vi "Acquisition State Machine.vi"(0 "Acquire":bool, 5 "Frames to Acquire":u32, 7 "Line Scan":bool, 9 "Line Scan Height":u32, 11 "Cancel Acq":bool, 12 "Enables":T1={"Enables Valid"=FALSE, "Frame Valid"=FALSE, "Line Valid"=FALSE, "Data Valid"=TRUE}) -> (4 "Acq In Progress":bool, 6 "Num Clocks Per Line":u32, 8 "Num Lines Per Frame":u32, 10 "Num Frames Acq'd":u32, 14 "Acquiring":bool, 15 "Capture Cycle":bool)   [LabVIEW 2014]
doc: "The Acquisition State Machine VI monitors its acquisition control inputs and tracks the state of the Camera Link enable signals to determine when pixel data should be captured and when it should be ignored, as indicated by the <B>Capture Cycle</B> output. The VI supports finite and continuous acquisitions for both area and line scan cameras. This VI is intended to run within a single-cycle timed loop.\n\nNote that the <B>Capture Cycle</B> output is delayed by two clock cycles relative to the <B>Enables</B> input. Also, this VI does not support cameras that change FVAL while LVAL is asserted. However, FVAL and LVAL are allowed to change at the same time. Open the VI for more documentation."
panel:
  # "Refer to the Context Help for a\ndescription of the controls and\nindicators of this VI."
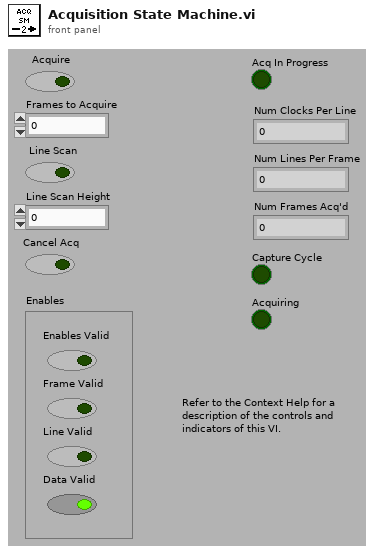
[diagram p1: front panel]
types:
  T1 = cluster{"Enables Valid":bool, "Frame Valid":bool, "Line Valid":bool, "Data Valid":bool}
  T2 = enum16{"Idle", "WaitForBlanking", "WaitForStartOfFrame", "WaitForEndOfFrame"}
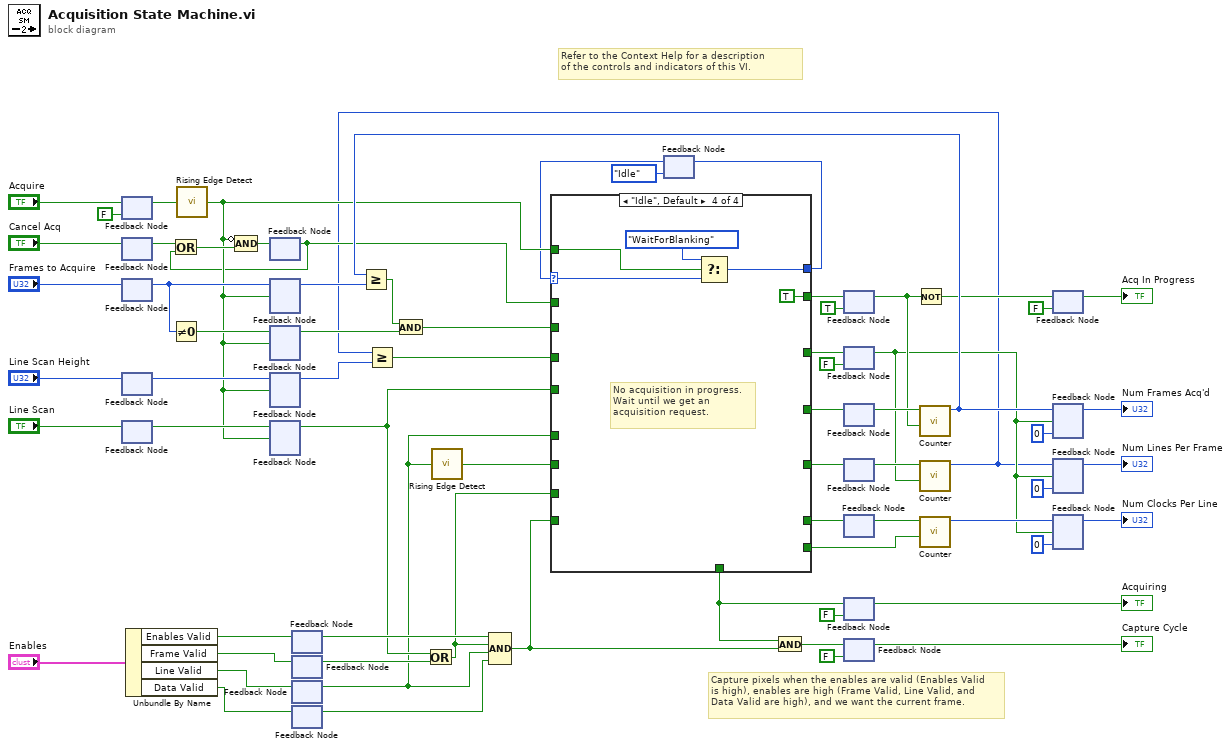
[diagram p0: block diagram]
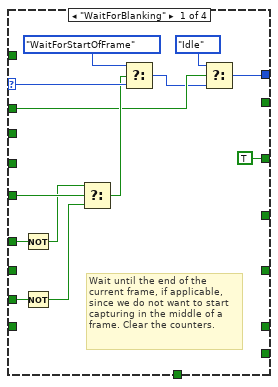
[diagram p2: hidden frame]
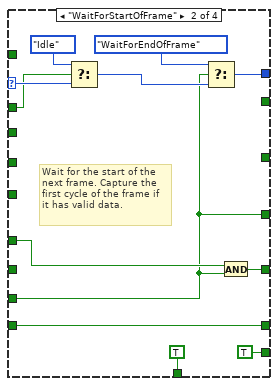
[diagram p3: hidden frame]
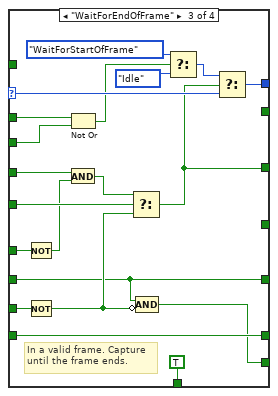
[diagram p4: hidden frame]
diagram:
  # "Refer to the Context Help for a description\nof the controls and indicators of this VI."
  # "Capture pixels when the enables are valid (Enables Valid\nis high), enables are high (Frame Valid, Line Valid, and\nData Valid are high), and we want the current frame."
  n1 = feedback #1(FALSE ("Acquire")) -> (w39:bool)
  n2 = feedback-in #1("Acquire") -> ()
  n3 = feedback #2() -> (w41:bool)  [unwired: 1 in]
  n4 = feedback-in #2("Cancel Acq") -> ()
  n5 = feedback #3() -> (w51:u32)  [unwired: 1 in]
  n6 = feedback-in #3("Frames to Acquire") -> ()
  n7 = feedback #4() -> (w36:u32)  [unwired: 1 in]
  n8 = feedback-in #4("Line Scan Height") -> ()
  n9 = feedback #5() -> (w34:bool)  [unwired: 1 in]
  n10 = feedback-in #5("Line Scan") -> ()
  n11 = Unbundle By Name("Enables") -> ("Enables Valid"=w29:bool, "Frame Valid"=w28:bool, "Line Valid"=w27:bool, "Data Valid"=w26:bool)
  n12 = Not Equal To 0?(x=w51) -> (x != 0?=w63:bool)
  n13 = call "Rising Edge Detect.vi"("Input"=w39) -> ("Pulse"=w33:bool)  [unwired: 4 in]
  n14 = feedback #6() -> (w25:bool)  [unwired: 1 in]
  n15 = Or(x=w41, y=w25) -> (x .or. y?=w43:bool)
  n16 = Compound Arithmetic op=AND(invert w33, w43) -> (w42:bool)
  n17 = feedback-in #6(w42) -> ()
  n18 = feedback #7() -> (w59:u32)  [unwired: 1 in]
  n19 = feedback-in #7(w51, w33) -> ()
  n20 = feedback #8() -> (w60:bool)  [unwired: 1 in]
  n21 = feedback-in #8(w63, w33) -> ()
  n22 = feedback #9() -> (w17:u32)  [unwired: 1 in]
  n23 = feedback-in #9(w36, w33) -> ()
  n24 = feedback #10() -> (w19:bool)  [unwired: 1 in]
  n25 = feedback-in #10(w34, w33) -> ()
  n26 = feedback #11() -> (w48:bool)  [unwired: 1 in]
  n27 = feedback-in #11(w29) -> ()
  n28 = feedback #12() -> (w32:bool)  [unwired: 1 in]
  n29 = feedback-in #12(w28) -> ()
  n30 = feedback #13() -> (w16:bool)  [unwired: 1 in]
  n31 = feedback-in #13(w27) -> ()
  n32 = feedback #14() -> (w46:bool)  [unwired: 1 in]
  n33 = feedback-in #14(w26) -> ()
  n34 = Or(x=w19, y=w32) -> (x .or. y?=w31:bool)
  n35 = call "Rising Edge Detect.vi"("Input"=w16) -> ("Pulse"=w40:bool)  [unwired: 4 in]
  n36 = Compound Arithmetic op=AND(w48, w31, w16, w46) -> (w47:bool)
  n37 = feedback #15(T2."Idle") -> (w23:T2)
  n38 = feedback #16(TRUE) -> (w20:bool)
  n39 = feedback #17(FALSE) -> (w6:bool)
  n40 = feedback #18() -> (w67:bool)  [unwired: 1 in]
  n41 = feedback #19() -> (w68:bool)  [unwired: 1 in]
  n42 = feedback #20() -> (w55:bool)  [unwired: 1 in]
  n43 = feedback #21(FALSE) -> (→"Acquiring":bool)
  n44 = feedback #22(FALSE) -> (→"Capture Cycle":bool)
  n45 = Not(x=w20) -> (.not. x?=w21:bool)
  n46 = call "Counter.vi"("Restart?"=w20, "Increment?"=w67) -> ("Count"=w62:u32)  [unwired: 9 in]
  n47 = Greater Or Equal?(x=w62, y=w59) -> (x >= y?=w61:bool)
  n48 = And(x=w61, y=w60) -> (x .and. y?=w18:bool)
  n49 = call "Counter.vi"("Restart?"=w6, "Increment?"=w68) -> ("Count"=w1:u32)  [unwired: 9 in]
  n50 = Greater Or Equal?(x=w1, y=w17) -> (x >= y?=w5:bool)
  n51 = case shown="\"Idle\", Default" w23 {
    selector: w23 -> [w82 w94 w113 w118]
    tunnel: [w75 w90 w114 w119] -> w22
    tunnel: [_ TRUE TRUE _] -> w3
    tunnel: w33 -> [_ _ _ w117]
    tunnel: w31 -> [w80 w83 w98 _]
    tunnel: [_ w85 w95 _] -> w69
    tunnel: [_ w83 _ _] -> w66
    tunnel: [TRUE _ w109 _] -> w8
    tunnel: w18 -> [_ _ w100 _]
    tunnel: [_ _ _ TRUE] -> w58
    tunnel: [_ w86 w111 _] -> w54
    tunnel: w47 -> [_ w86 w111 _]
    tunnel: [_ TRUE w97 _] -> w53
    tunnel: w40 -> [_ _ w95 _]
    tunnel: w5 -> [_ _ w102 _]
    tunnel: w19 -> [w81 _ w106 _]
    tunnel: w25 -> [w77 w89 w101 _]
    tunnel: w16 -> [w72 w84 w105 _]
    frame "WaitForBlanking" {
      # "Wait until the end of the\ncurrent frame, if applicable,\nsince we do not want to start\ncapturing in the middle of a\nframe. Clear the counters."
      n52 = Not(x=w72) -> (.not. x?=w71:bool)
      n53 = Not(x=w80) -> (.not. x?=w78:bool)
      n54 = Select(t=w71, s=w81, f=w78) -> (s? t:f=w79:bool)
      n55 = Select(t=T2."WaitForStartOfFrame", s=w79, f=w82) -> (s? t:f=w76:T2)
      n56 = Select(t=T2."Idle", s=w77, f=w76) -> (s? t:f=w75:T2)
    }
    frame "WaitForStartOfFrame" {
      # "Wait for the start of the\nnext frame. Capture the\nfirst cycle of the frame if\nit has valid data."
      n57 = Select(t=T2."Idle", s=w89, f=w94) -> (s? t:f=w91:T2)
      n58 = Select(t=T2."WaitForEndOfFrame", s=w83, f=w91) -> (s? t:f=w90:T2)
      n59 = And(x=w84, y=w83) -> (x .and. y?=w85:bool)
    }
    frame "WaitForEndOfFrame" {
      # "In a valid frame. Capture\nuntil the frame ends."
      n60 = Not(x=w105) -> (.not. x?=w104:bool)
      n61 = Not(x=w98) -> (.not. x?=w96:bool)
      n62 = Not Or(1:w100, 2:w101) -> (0:w99:bool)
      n63 = And(x=w102, y=w104) -> (x .and. y?=w103:bool)
      n64 = Select(t=w103, s=w106, f=w96) -> (s? t:f=w109:bool)
      n65 = Compound Arithmetic op=AND(w95, invert w96) -> (w97:bool)
      n66 = Select(t=T2."WaitForStartOfFrame", s=w99, f=T2."Idle") -> (s? t:f=w110:T2)
      n67 = Select(t=w110, s=w109, f=w113) -> (s? t:f=w114:T2)
    }
    frame "Idle", Default {
      # "No acquisition in progress.\nWait until we get an\nacquisition request."
      n68 = Select(t=T2."WaitForBlanking", s=w117, f=w118) -> (s? t:f=w119:T2)
    }
  }
  n69 = feedback-in #15(w22) -> ()
  n70 = And(x=w3, y=w47) -> (x .and. y?=w45:bool)
  n71 = feedback-in #16(w58) -> ()
  n72 = feedback-in #17(w8) -> ()
  n73 = feedback-in #18(w66) -> ()
  n74 = feedback-in #19(w69) -> ()
  n75 = feedback-in #20(w54) -> ()
  n76 = feedback-in #21(w3) -> ()
  n77 = feedback-in #22(w45) -> ()
  n78 = call "Counter.vi"("Restart?"=w53, "Increment?"=w55) -> ("Count"=w56:u32)  [unwired: 9 in]
  n79 = feedback #23(FALSE) -> (→"Acq In Progress":bool)
  n80 = feedback-in #23(w21) -> ()
  n81 = feedback #24(u32 0 ("Count")) -> (→"Num Frames Acq'd":u32)
  n82 = feedback-in #24(w62, w6) -> ()
  n83 = feedback #25(u32 0) -> (→"Num Lines Per Frame":u32)
  n84 = feedback-in #25(w1, w6) -> ()
  n85 = feedback #26(u32 0 ("Count")) -> (→"Num Clocks Per Line":u32)
  n86 = feedback-in #26(w56, w6) -> ()
